vi "IAmGLF-CreateDVR.vi"(8 "error in (no error)":errorcluster, 11 "View in":refnum<class "View.lvclass">) -> (0 "error out":errorcluster, 3 "View out":refnum<class "View.lvclass">)   [LabVIEW 2024, in "GLF.lvlib" / "View.lvclass"]
doc: "<B>Summary</B>\nTo create the class DVR in an standalone process."
uses:
  View.lvclass
  DVR--cluster.ctl
  View.lvclass/View.ctl
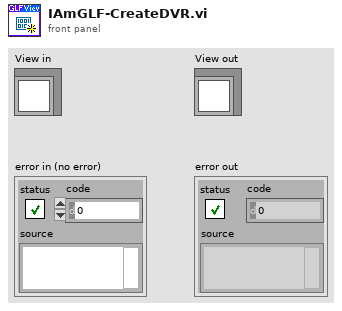
[diagram p1: front panel]
types:
  T1 = typedef "GLF.lvlib/View.lvclass/DVR--cluster.ctl" = cluster{"foo":dbl}
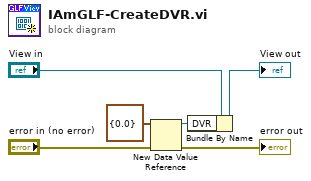
[diagram p0: block diagram]
diagram:
  n1 = New Data Value Reference(data value=T1 {"foo"=0.0} ("DVR"), error in="error in (no error)") -> (data value reference=w3:refnum<data-value>, error out=→"error out":errorcluster)
  n2 = Bundle By Name(cluster="View in", "DVR"=w3) -> (→"View out":refnum<class "View.lvclass">)
